vi "plot band positions.vi"(4 "band":i16, 5 "total bands":i16, 7 "Draw Area Size":cluster{"Width":u32, "Height":u32}) -> (0 "bottom":u32, 1 "top":u32, 3 "band positions":cluster{"top":u32, "bottom":u32}[](array[cluster]))   [LabVIEW 2012]
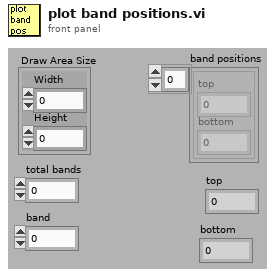
[diagram p1: front panel]
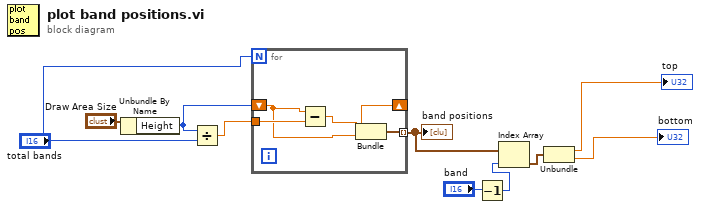
[diagram p0: block diagram]
diagram:
  n1 = Unbundle By Name("Draw Area Size") -> ("Height"=w8:u32)
  n2 = Divide(x=w8, y="total bands") -> (x/y=w7:dbl)
  n3 = for {
    N: "total bands" -> [_]
    shift-right: [w13] -> _
    shift-left: w8 -> [w12]
    tunnel: w7 -> [w14]
    tunnel: [w11] -> w6 mode=indexing
    n4 = Subtract(x=w12, y=w14) -> (x-y=w13:dbl)
    n5 = Bundle(w13, "Height"=w12) -> (w11:cluster{dbl, "Height":dbl})  [unwired: 1 in]
  }
  "band positions" <- w6
  n6 = Decrement(x="band") -> (x-1=w1:i16)
  n7 = Index Array(array=w6, index=w1) -> (element=w5:cluster{dbl, "Height":dbl})
  n8 = Unbundle(w5) -> (→"top":dbl, "Height"=→"bottom":dbl)
